vi "RiversideRelayReadChannel.vi"(0 "serial_number":string="Z8KHE", 1 "Relay Channel":i32=1, 3 "error in":errorcluster) -> (5 "Transducer":enum16{"Transducer 1", "Transducer 2"}(ring), 7 "error out":errorcluster)   [LabVIEW 2022 SP3]
uses:
  SwitchGlobals.vi
  usb_relay_device/usb_relay_device.lvlib
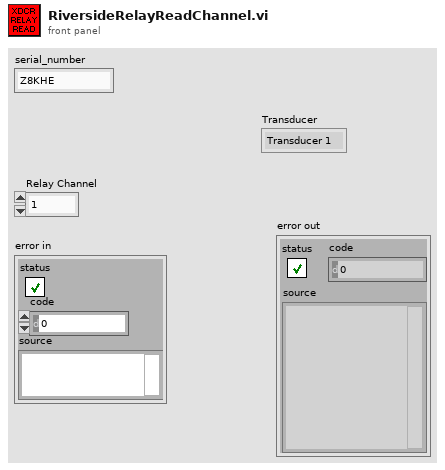
[diagram p1: front panel]
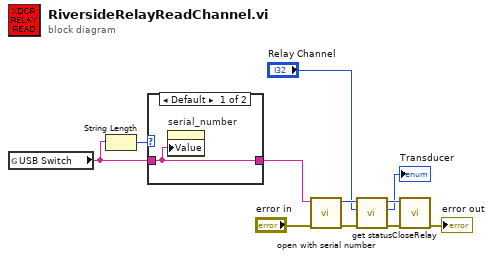
[diagram p0: block diagram]
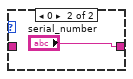
[diagram p2: hidden frame]
diagram:
  n1 = global read "SwitchGlobals.vi" "USB Switch"() -> (w2:string)
  n2 = String Length(string=w2) -> (length=w3:i32)
  n3 = case shown="Default" w3 {
    tunnel: [w12 "serial_number"] -> w1
    tunnel: w2 -> [w12 _]
    frame Default {
      n4 = property on="serial_number" class="Str"("Value"=w12) -> ()  [unwired: 2 in, 2 out]
    }
    frame 0 {
    }
  }
  n5 = call "open with serial number.vi"("error in (no error)"="error in", "serial_number"=w1) -> ("error out"=w6:errorcluster, "Relay Identifier"=w9:i32)  [unwired: 8 in]
  n6 = call "get status.vi"("error in (no error)"=w6, "status"="Relay Channel", "Relay Indetifier"=w9) -> ("error out"=w7:errorcluster, "status out"=→"Transducer":u32, "Relay Indetifier Out"=w8:i32)  [unwired: 6 in]
  n7 = call "CloseRelay.vi"("error in (no error)"=w7, "Relay Identifier"=w8) -> ("error out"=→"error out":errorcluster)  [unwired: 9 in]
